vi "ReadAndWriteFile.vi"(11 "String":string) -> (3 "data out":string)   [LabVIEW 2020]
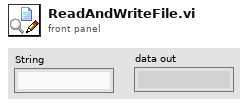
[diagram p1: front panel]
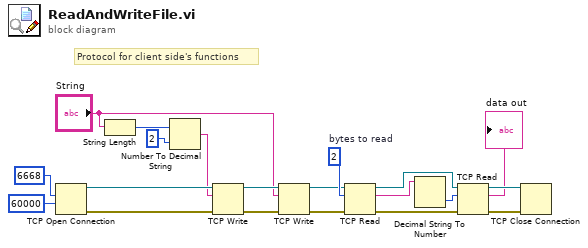
[diagram p0: block diagram]
diagram:
  w17 = 2  # bytes to read
  # "Protocol for client side's functions"
  n1 = TCP Open Connection(remote port or service name=u16 6668, timeout ms (60000)=60000) -> (connection ID=w16:refnum<k5>, error out=w7:errorcluster)  [unwired: 3 in]
  n2 = String Length(string="String") -> (length=w6:i32)
  n3 = Number To Decimal String(number=w6, width (-)=i16 2) -> (decimal integer string=w5:string)
  n4 = TCP Write(connection ID=w16, data in=w5, error in (no error)=w7) -> (connection ID out=w15:refnum<k5>, error out=w8:errorcluster)  [unwired: 1 in, 1 out]
  n5 = TCP Write(connection ID=w15, data in="String", error in (no error)=w8) -> (connection ID out=w14:refnum<k5>, error out=w9:errorcluster)  [unwired: 1 in, 1 out]
  n6 = TCP Read(connection ID=w14, bytes to read=w17, error in (no error)=w9) -> (connection ID out=w13:refnum<k5>, data out=w3:string, error out=w10:errorcluster)  [unwired: 2 in]
  n7 = Decimal String To Number(string=w3) -> (number=w2:i32)  [unwired: 2 in, 1 out]
  n8 = TCP Read(connection ID=w13, bytes to read=w2, error in (no error)=w10) -> (connection ID out=w12:refnum<k5>, data out=→"data out":string, error out=w11:errorcluster)  [unwired: 2 in]
  n9 = TCP Close Connection(connection ID=w12, error in (no error)=w11) -> ()  [unwired: 1 in, 2 out]
